vi "RT Error Handler - Watchdog.vi"(8 "error in (no error)":errorcluster, 10 "watchdog status":T1, 11 "Message Queue":refnum<queue>) -> (3 "dup Message Queue":refnum<queue>)   [LabVIEW 2018]
uses:
  Support/Message Queue/Message Cluster.ctl
  Support/Message Queue/Message.ctl
  <vilib>/RTwatchdog.llb/Watchdog status enum.ctl
  support/Message Queue/Message Queue.lvlib
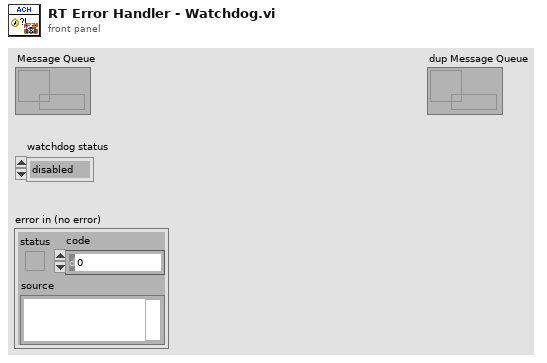
[diagram p1: front panel]
types:
  T1 = typedef "Watchdog status enum.ctl" = enum16{"disabled", "expired", "running"}
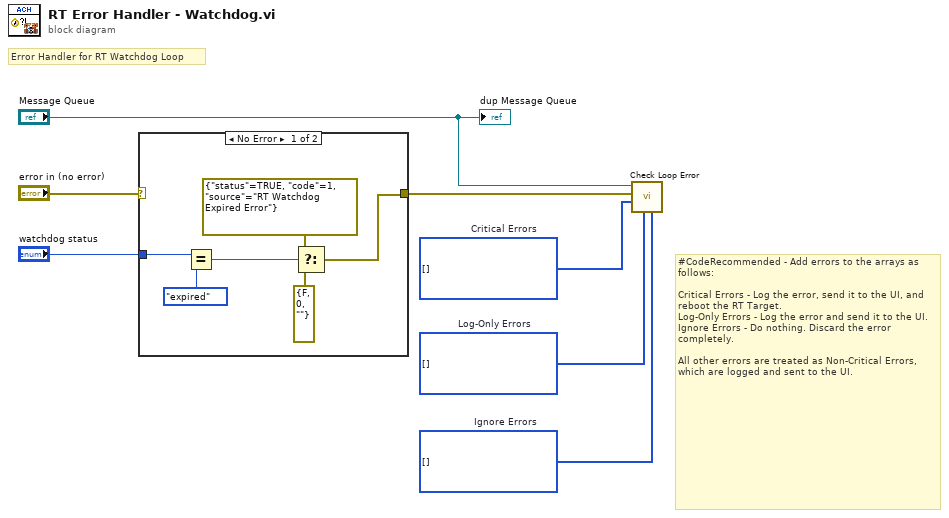
[diagram p0: block diagram]
diagram:
  w5 = i32[] []  # Ignore Errors
  w6 = i32[] []  # Log-Only Errors
  w7 = i32[] []  # Critical Errors
  # "#CodeRecommended - Add errors to the arrays as follows:\n\nCritical Errors - Log the error, send it to the UI, and reboot the RT Target.\nLog-Only Errors - Log the error and send it to the UI.\nIgnore Errors - Do nothing. Discard the error completely.\n\nAll other errors are treated as Non-Critical Errors, which are logged and sent to the UI."
  # "Error Handler for RT Watchdog Loop"
  n1 = case shown="No Error" "error in (no error)" {
    selector: "error in (no error)" -> [_ w14]
    tunnel: [w9 w14] -> w2
    tunnel: "watchdog status" -> [w13 _]
    frame No Error {
      n2 = Equal?(x=w13, y=Watchdog_status_enum."expired") -> (x = y?=w11:bool)
      n3 = Select(t=errorcluster {"status"=TRUE, "code"=1, "source"="RT Watchdog Expired Error"} ("error constant"), s=w11, f=errorcluster {"status"=FALSE, "code"=0, "source"=""} ("error constant")) -> (s? t:f=w9:errorcluster)
    }
    frame Error {
    }
  }
  n4 = call "Check Loop Error.vi"("Ignore Errors"=w5, "Log-Only Errors"=w6, "Critical Errors"=w7, "error to process"=w2, "Message Queue"="Message Queue") -> ()  [unwired: 5 in, 2 out]
  "dup Message Queue" <- "Message Queue"
